vi "GetBorders.vi"(8 "error in (no error)":errorcluster, 11 "path to PNG file":path) -> (0 "error out":errorcluster, 6 "Borders":cluster{dbl}[](array[cluster]))   [LabVIEW 2022 SP3]
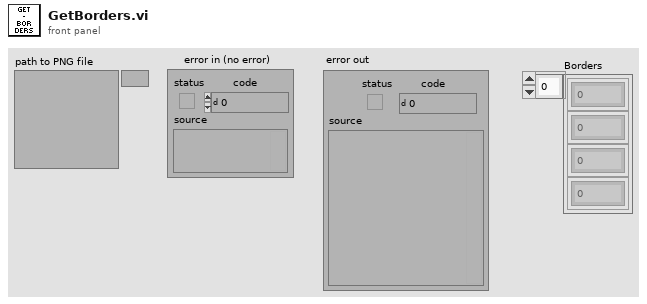
[diagram p1: front panel]
types:
  T1 = typedef "imagedata.ctl" = cluster{"image type":i32, "image depth":i32, "image":u8[], "mask":u8[], "colors":u32[], "Rectangle":cluster{"left":i16, "top":i16, "right":i16, "bottom":i16}}
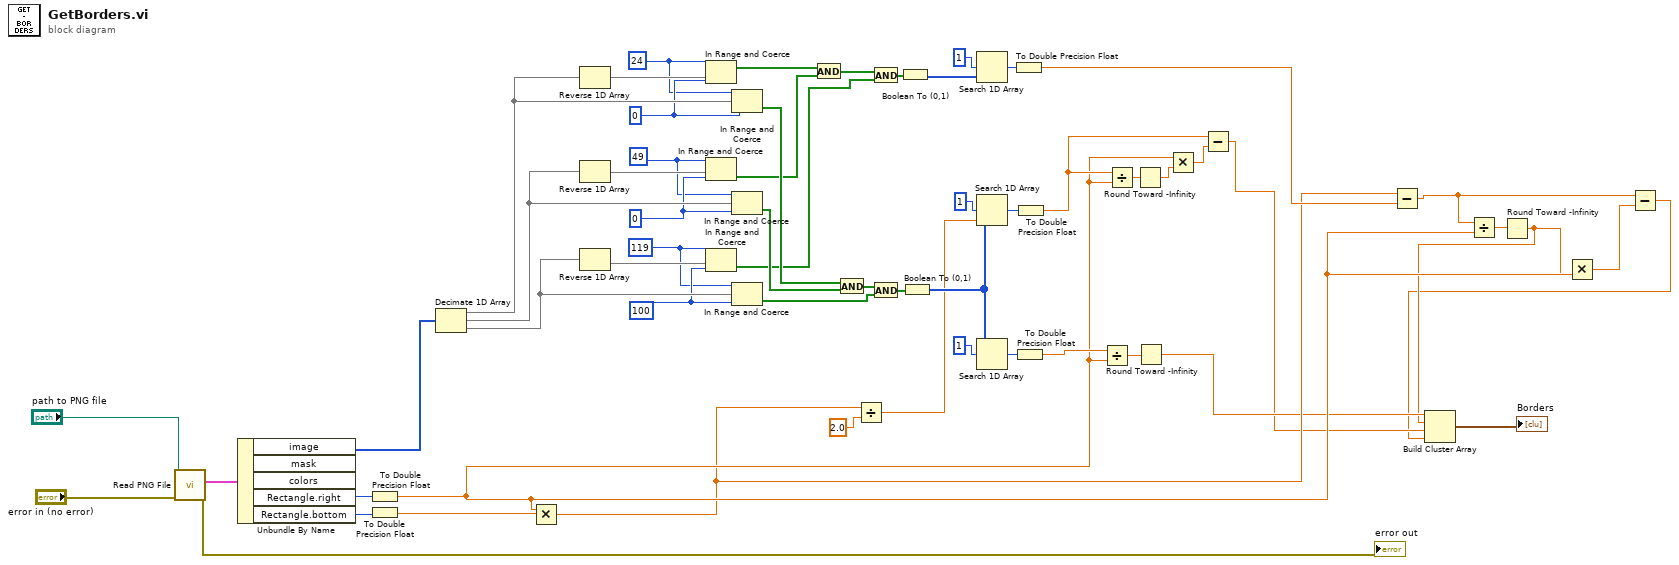
[diagram p0: block diagram]
diagram:
  w19 = u8 100 ("B min")
  w18 = u8 119 ("B max")
  w17 = u8 0 ("G min")
  w16 = u8 49 ("G max")
  w15 = u8 0 ("R min")
  w14 = u8 24 ("R max")
  n1 = call <vilib>:"Read PNG File.vi"("error in (no error)"="error in (no error)", "path to PNG file"="path to PNG file") -> ("error out"=→"error out":errorcluster, "image data"=w57:T1)  [unwired: 7 in, 1 out]
  n2 = Unbundle By Name(w57) -> ("image"=w1:u8[], "Rectangle.right"=w47:i16, "Rectangle.bottom"=w46:i16)  [unwired: 2 out]
  n3 = To Double Precision Float(number=w47) -> (double precision float=w13:dbl)
  n4 = To Double Precision Float(number=w46) -> (double precision float=w45:dbl)
  n5 = Decimate 1D Array "Decimate 1D Array"(w1) -> (w30:u8[], w29:u8[], w28:u8[])
  n6 = Multiply(x=w13, y=w45) -> (x*y=w12:dbl)
  n7 = Reverse 1D Array(array=w30) -> (reversed array=w24:u8[])
  n8 = Reverse 1D Array(array=w29) -> (reversed array=w25:u8[])
  n9 = Reverse 1D Array(array=w28) -> (reversed array=w23:u8[])
  n10 = In Range and Coerce(upper limit=w14, x=w24, lower limit=w15) -> (In Range?=w26:bool[])  [unwired: 1 out]
  n11 = In Range and Coerce(upper limit=w16, x=w25, lower limit=w17) -> (In Range?=w27:bool[])  [unwired: 1 out]
  n12 = In Range and Coerce(upper limit=w18, x=w23, lower limit=w19) -> (In Range?=w22:bool[])  [unwired: 1 out]
  n13 = In Range and Coerce(upper limit=w14, x=w30, lower limit=w15) -> (In Range?=w52:bool[])  [unwired: 1 out]
  n14 = In Range and Coerce(upper limit=w16, x=w29, lower limit=w17) -> (In Range?=w53:bool[])  [unwired: 1 out]
  n15 = In Range and Coerce(upper limit=w18, x=w28, lower limit=w19) -> (In Range?=w54:bool[])  [unwired: 1 out]
  n16 = And(x=w26, y=w27) -> (x .and. y?=w21:bool[])
  n17 = And(x=w52, y=w53) -> (x .and. y?=w51:bool[])
  n18 = Divide(x=w12, y=2.0) -> (x/y=w31:dbl)
  n19 = And(x=w21, y=w22) -> (x .and. y?=w49:bool[])
  n20 = And(x=w51, y=w54) -> (x .and. y?=w55:bool[])
  n21 = Boolean To (0,1)(Boolean=w49) -> (0, 1=w50:i16[])
  n22 = Boolean To (0,1)(Boolean=w55) -> (0, 1=w32:i16[])
  n23 = Search 1D Array(1D array=w50, element=i16 1) -> (index of element=w48:i32)  [unwired: 1 in]
  n24 = Search 1D Array(1D array=w32, element=i16 1, start index (0)=w31) -> (index of element=w38:i32)
  n25 = Search 1D Array(1D array=w32, element=i16 1) -> (index of element=w43:i32)  [unwired: 1 in]
  n26 = To Double Precision Float(number=w48) -> (double precision float=w44:dbl)
  n27 = To Double Precision Float(number=w43) -> (double precision float=w42:dbl)
  n28 = To Double Precision Float(number=w38) -> (double precision float=w34:dbl)
  n29 = Divide(x=w42, y=w13) -> (x/y=w41:dbl)
  n30 = Divide(x=w34, y=w13) -> (x/y=w37:dbl)
  n31 = Round Toward -Infinity(1:w37) -> (0:w36:dbl)
  n32 = Round Toward -Infinity(1:w41) -> (0:w5:dbl)
  n33 = Multiply(x=w13, y=w36) -> (x*y=w35:dbl)
  n34 = Subtract(x=w34, y=w35) -> (x-y=w3:dbl)
  n35 = Subtract(x=w12, y=w44) -> (x-y=w20:dbl)
  n36 = Divide(x=w20, y=w13) -> (x/y=w33:dbl)
  n37 = Round Toward -Infinity(1:w33) -> (0:w4:dbl)
  n38 = Multiply(x=w13, y=w4) -> (x*y=w40:dbl)
  n39 = Subtract(x=w20, y=w40) -> (x-y=w2:dbl)
  n40 = Build Cluster Array(w5, w4, w3, w2) -> (→"Borders":cluster{dbl}[])
